vi "Update_GeneratedFiles_Preview.vi"(8 "error in (no error)":errorcluster, 9 "GeneratedFiles in":path[](array[path]), 10 "GeneratedFileGUIDs in":string[](array[string]), 11 "Build in":refnum<class "AB_WebService.lvclass">) -> (0 "error out":errorcluster, 1 "GeneratedFiles out":path[](array[path]), 2 "GeneratedFileGUIDs out":string[](array[string]), 3 "Build out":refnum<class "AB_WebService.lvclass">)   [LabVIEW 2020, in "AB_WebService.lvclass"]
uses:
  <vilib>/AppBuilder/AB_Classes/WebService/AB_WebService.lvclass
  e:/builds/penguin/labview/branches/2020/dev/dist/vi.lib/AppBuilder/AB_Classes/Build/AB_Build.lvclass
  e:/builds/penguin/labview/branches/2020/dev/dist/vi.lib/AppBuilder/AB_Classes/TargetFile/AB_Targetfile.lvclass
  <vilib>/AppBuilder/AB_Classes/Destination/AB_Destination.lvclass
  <vilib>/AppBuilder/AB_Classes/Build/AB_Build.lvclass
  <vilib>/AppBuilder/AB_Classes/TargetFile/AB_Targetfile.lvclass
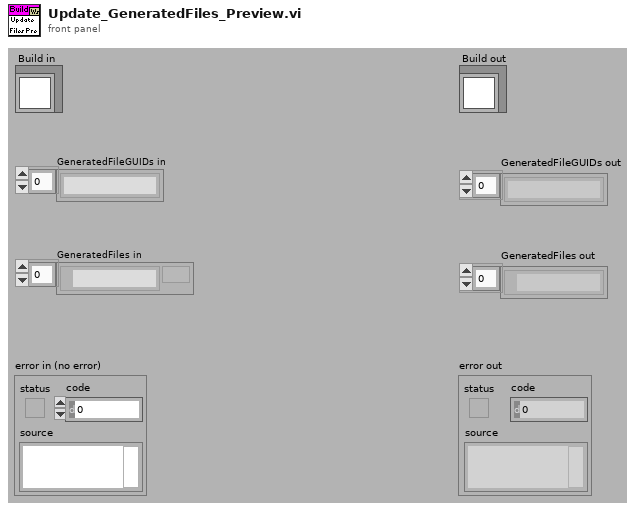
[diagram p1: front panel]
types:
  T1 = typedef "AB_Build.ctl" = cluster{"buildSpecName":string, "buildSpecDescription":string, "destinations":refnum<class "AB_Destination.lvclass">[], "exclusionOption":T2, "defaultLanguage":string, "supportedLanguages":string[], "excludedDirectories":path[], "buildContext":refnum<vi>, "buildObject":T3, "preview":bool, "programatic":bool, "progressBarEvents":T4, "userLog_Path":path, "preActionID":string, "preAction_Path":path, "postActionID":string, "postAction_Path":path, "eng_checkForBrokenVIs?":bool, "eng_verboseLinkerErrors?":bool, "localDest_Path":path, "targetDest_Path":path, "removeVIObject":u16, "cache":refnum<class "PreviewCache.lvclass">, "use cache":bool, "previewCache_ID":string, "buildCache_ID":string, "eng_TempLocalDest_Path":path, "eng_collectDependencies?":bool, "versionInfo":cluster{"buildVersion":cluster{"major":u16, "minor":u16, "patch":u16, "build":u16}, "autoIncrement":bool}, "eng_enableVIChecksums":bool}
  T2 = typedef "AB_Exclusion_Option.ctl" = cluster{"typedefs":bool, "polymorphicVIs":bool, "unusedLibraryItems":bool, "modifyLibraryFile":bool, "edit-timeDependencies":bool, "inlineVIs":bool, "dependent PPLs":bool, "dependent DLLs":bool}
  T3 = typedef "ItemRef.ctl" = u64
  T4 = typedef "provcom_ProgressBar_Events.ctl" = cluster{"newJob":refnum<user-event>, "newItem":refnum<user-event>, "errorMsg":T5, "cancel":refnum<user-event>}
  T5 = typedef "mxLvBuildError.ctl" = refnum<user-event>
  T6 = typedef "AB_Targetfile.ctl" = cluster{"targetfileName":string, "targetfileGUID":string, "enableDebugging":bool, "versionInfo":cluster{"productName":string, "legalCopyright":string, "companyName":string, "internalName":string, "fileDescription":string}, "eng_consolidatedTypeInfo":string, "fastFileFormat":bool, "eng_LEIFBuildData":u32, "versionIndependent":bool}
  T7 = typedef "AB_Destination.ctl" = cluster{"destName":string, "path":path, "libraryName":string, "preserveHierarchy":bool, "eng_inBuild":bool, "eng_libraryReference":refnum<vi>, "eng_restictAddToNewLibrary":bool}
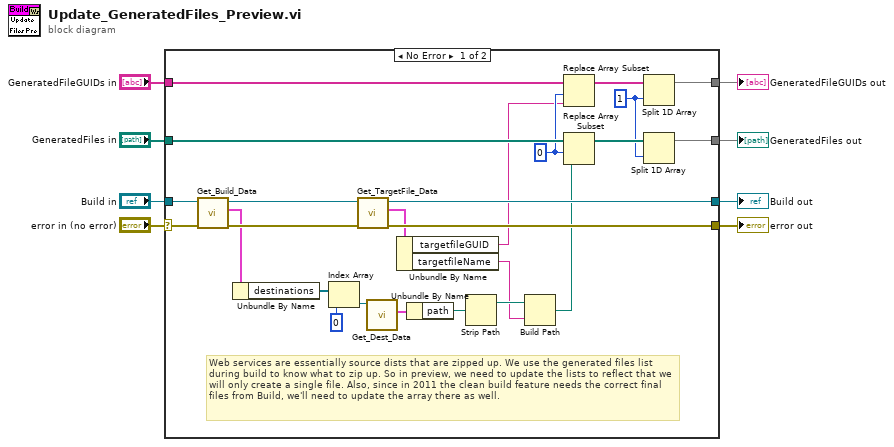
[diagram p0: block diagram]
diagram:
  n1 = case shown="No Error" "error in (no error)" {
    selector: "error in (no error)" -> [w9 w36]
    tunnel: [w29 w36] -> w8
    tunnel: "Build in" -> [w10 w37]
    tunnel: [w28 w37] -> w7
    tunnel: "GeneratedFileGUIDs in" -> [w32 w34]
    tunnel: "GeneratedFiles in" -> [w33 w35]
    tunnel: [w30 w35] -> w6
    tunnel: [w31 w34] -> w5
    frame No Error {
      w17 = 1 ("index")
      w23 = 0 ("index")
      # "Web services are essentially source dists that are zipped up. We use the generated files list during build to know what to zip up. So in preview, we need to update the lists to reflect that we will only create a single file. Also, since in 2011 the clean build feature needs the correct final files from Build, we'll need to update the array there as well."
      n2 = call <vilib>:"Get_Build_Data.vi"("error in (no error)"=w9, "Class in"=w10) -> ("error out"=w13:errorcluster, "data"=w12:T1, "Class out"=w14:refnum<class "AB_WebService.lvclass">)  [unwired: 7 out]
      n3 = Unbundle By Name(w12) -> ("destinations"=w11:refnum<class "AB_Destination.lvclass">[])
      n4 = Index Array(array=w11, index=0) -> (element=w26:refnum<class "AB_Destination.lvclass">)
      n5 = call <vilib>:"Get_TargetFile_Data.vi"("error in (no error)"=w13, "AB_Targetfile in"=w14) -> ("error out"=w29:errorcluster, "data"=w16:T6, "AB_Targetfile out"=w28:refnum<class "AB_WebService.lvclass">)  [unwired: 7 in]
      n6 = call <vilib>:"Get_Dest_Data.vi"("Class in"=w26) -> ("destName"=w25:T7)  [unwired: 1 in, 9 out]
      n7 = Unbundle By Name(w16) -> ("targetfileGUID"=w22:string, "targetfileName"=w15:string)
      n8 = Unbundle By Name(w25) -> ("path"=w27:path)
      n9 = Strip Path(path=w27) -> (stripped path=w21:path)  [unwired: 1 out]
      n10 = Build Path(base path=w21, name or relative path=w15) -> (appended path=w20:path)
      n11 = Replace Array Subset(array=w32, new element=w22, index=w23) -> (w19:string[])
      n12 = Replace Array Subset(array=w33, new element=w20, index=w23) -> (w18:path[])
      n13 = Split 1D Array(array=w19, index=w17) -> (first subarray=w31:string[])  [unwired: 1 out]
      n14 = Split 1D Array(array=w18, index=w17) -> (first subarray=w30:path[])  [unwired: 1 out]
    }
    frame Error {
    }
  }
  "error out" <- w8
  "Build out" <- w7
  "GeneratedFiles out" <- w6
  "GeneratedFileGUIDs out" <- w5
